vi "Test NI-Scope Performance.vi"() -> ()   [LabVIEW 2016]
uses:
  NI-Scope Lock-in Driver/NI-Scope Lock-in Configuration.ctl
  Instruments/Temperature Controller Driver/T controller configuration.ctl
  NI-Scope Lock-in Driver/NI-Scope Lock-in Driver.lvclass
  C:/github/NHMFL_Core/Libraries/Instruments/Pulse Driver/Pulse Driver.lvclass
  C:/github/NHMFL_Core/Libraries/NI-DAQ/NI-Scope Digitizer/Ni-Scope Digitizer.lvclass
  Instruments/Cryo-con/Cryo-Con Driver/Cryo-Con Driver.lvclass
  C:/github/NHMFL_Core/Libraries/Instruments/VISA Instrument/VISA Instrument.lvclass
  C:/github/NHMFL_Core/Libraries/Instruments/Temperature Controller Driver/Temperature Controller Driver.lvclass
  C:/github/NHMFL_Core/Libraries/Instruments/Instrument Driver/Instrument Driver.lvclass
  Instruments/Pulse Driver/Pulse Driver.lvclass/Pulse Driver.ctl
  Ni-Scope Digitizer.lvclass/Ni-Scope Digitizer.ctl
  Instruments/VISA Instrument/VISA Instrument.lvclass/VISA Instrument.ctl
  Instruments/Instrument Driver/Instrument Driver.lvclass/Instrument Driver.ctl
  Instruments/VISA Instrument/Write VISA resource.vi
  Instruments/Instrument Driver/Write Recorder name.vi
  Instruments/Pulse Driver/Write tdms file.vi
  Write Device name.vi
  Write Fetch Relative To.vi
  Instruments/Pulse Driver/Write Samples per read.vi
  Instruments/Temperature Controller Driver/Write T controller configuration.vi
  Instruments/Results/Acquired Result/Acquired Result.lvclass
panel:
  in  "T controller configuration":T1={"Record Channels"=["A"], "Add raw signal"=FALSE, "New set point"=0.0}
  in  "Cryocon VISA resource":refnum<visa-resource-name>="COM4"
  out "File Path Control":path
  out "Waveform Chart":dynamicdata(graph)
  in  "milliseconds to wait":u32=1000
  in  "Configuration":T2={"Points per sine wave"=64, "Rate"=4096012.1154785156, "Re-name channels"=["I", "Va", "Vc1", "Vc2"], "Active channels"="2", "Ranges"=[10.0], "Sync on trigger"=TRUE, "R-Q"=FALSE} {"Ranges" format="%#_6pV"; "Rate" format="%#_8pHz"}
  in  "Device name":refnum<k15>="5105-PCI"
  in  "Stop Button":bool
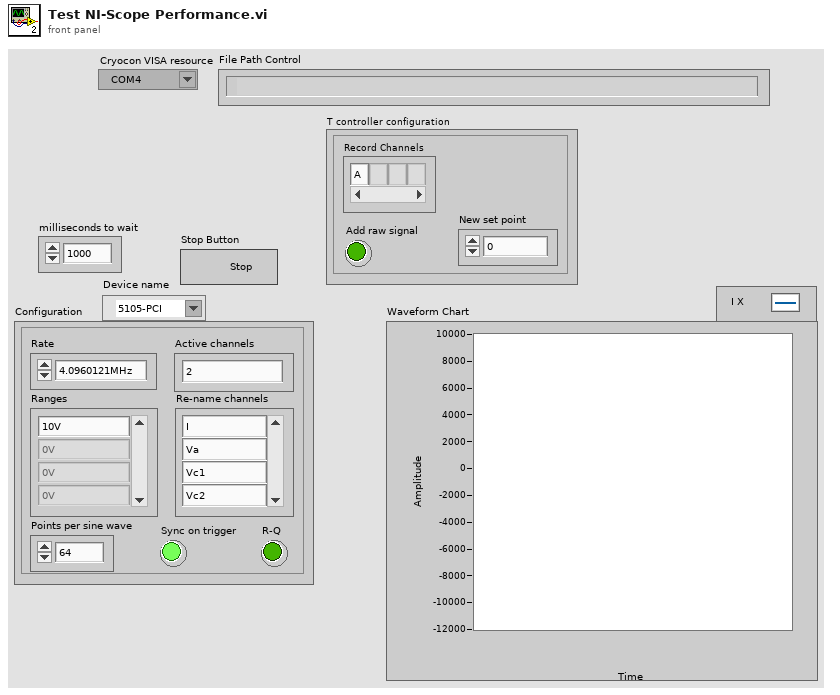
[diagram p1: front panel]
types:
  T1 = typedef "T controller configuration.ctl" = cluster{"Record Channels":string[], "Add raw signal":bool, "New set point":dbl}
  T2 = typedef "NI-Scope Lock-in Configuration.ctl" = cluster{"Points per sine wave":i32, "Rate":dbl, "Re-name channels":string[], "Active channels":string, "Ranges":dbl[], "Sync on trigger":bool, "R-Q":bool}
  T3 = enum16{"open", "open or create", "create or replace", "create", "open (read-only)"}
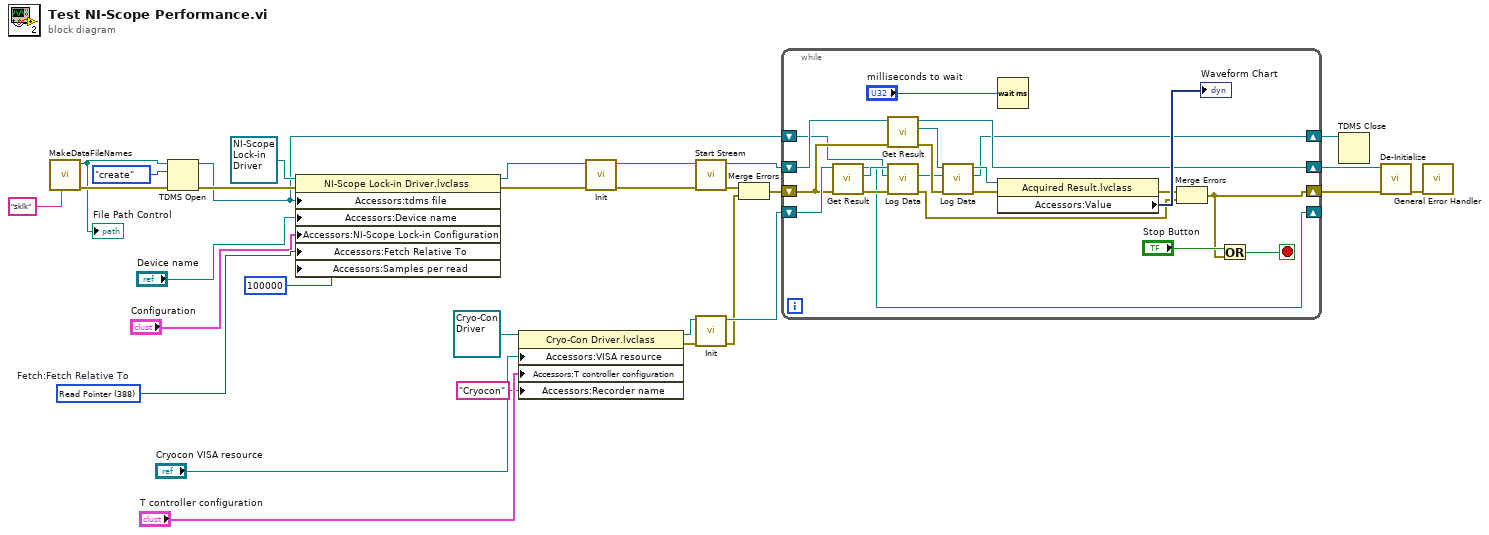
[diagram p0: block diagram]
diagram:
  w28 = 388 items=["Start"=482, "Trigger"=483, "Pretrigger"=477, "Now"=481, "Read Pointer"=388]  # Fetch:Fetch Relative To
  n1 = call "MakeDataFileNames.vi"("File Prefix"="sklk") -> ("Error Out"=w22:errorcluster, "Data File  Path"=w18:path)  [unwired: 7 in, 2 out]
  "File Path Control" <- w18
  n2 = TDMS Open(8:w22, 10:T3."create" ("operation (0:open)"), 11:w18) -> (0:w21:errorcluster, 3:w13:refnum<k34>)  [unwired: 4 in]
  n3 = property class="NI-Scope Lock-in Driver.lvclass"(reference=refnum<class "NI-Scope Lock-in Driver.lvclass"> refnum ("NI-Scope Lock-in Driver.lvclass"), error in=w21, "Accessors:tdms file"=w13, "Accessors:Device name"="Device name", "Accessors:NI-Scope Lock-in Configuration"="Configuration", "Accessors:Fetch Relative To"=w28, "Accessors:Samples per read"=100000 ("Samples per read")) -> (reference out=w29:refnum<class "NI-Scope Lock-in Driver.lvclass">, error out=w10:errorcluster)
  n4 = property class="Cryo-Con Driver.lvclass"(reference=refnum<class "Cryo-Con Driver.lvclass"> refnum ("Cryo-Con Driver.lvclass"), "Accessors:VISA resource"="Cryocon VISA resource", "Accessors:T controller configuration"="T controller configuration", "Accessors:Recorder name"="Cryocon" ("Recorder name")) -> (reference out=w6:refnum<class "Cryo-Con Driver.lvclass">, error out=w4:errorcluster)  [unwired: 1 in]
  n5 = call-dynamic "Init.vi"("error in (no error)"=w10, "Instrument Driver in"=w29) -> ("error out"=w15:errorcluster, "Instrument Driver out"=w17:refnum<class "NI-Scope Lock-in Driver.lvclass">)  [unwired: 7 in, 1 out]
  n6 = call-dynamic "Start Stream.vi"("error in (no error)"=w15, "Ni-Scope Digitizer in"=w17) -> ("error out"=w14:errorcluster, "Ni-Scope Digitizer out"=w16:refnum<class "NI-Scope Lock-in Driver.lvclass">)  [unwired: 8 in]
  n7 = call-dynamic "Init.vi"("error in (no error)"=w4, "Instrument Driver in"=w6) -> ("error out"=w3:errorcluster, "Instrument Driver out"=w5:refnum<class "Cryo-Con Driver.lvclass">)  [unwired: 7 in, 1 out]
  n8 = Merge Errors(w14, w3) -> (w9:errorcluster)
  n9 = while {
    shift-right: [w45] -> w26
    shift-left: w16 -> [w48]
    shift-right: [w31] -> w27
    shift-left: w9 -> [w39]
    shift-right: [w36] -> w8
    shift-left: w13 -> [w35]
    shift-right: [w32] -> _
    shift-left: w5 -> [w40]
    stop <- w49 stop-if-true
    n10 = call-dynamic "Get Result.vi"("error in (no error)"=w39, "Simple VISA Reader Driver in"=w40) -> ("error out"=w37:errorcluster, "Result"=w38:refnum<class "Acquired Result.lvclass">, "Simple VISA Reader Driver out"=w32:refnum<class "Cryo-Con Driver.lvclass">)  [unwired: 7 in]
    n11 = call-dynamic "Get Result.vi"("error in (no error)"=w39, "NI-Scope Lock-in Driver in"=w48) -> ("error out"=w43:errorcluster, "Result"=w44:refnum<class "Acquired Result.lvclass">, "NI-Scope Lock-in Driver out"=w45:refnum<class "NI-Scope Lock-in Driver.lvclass">)  [unwired: 7 in]
    n12 = call-dynamic "Log Data.vi"("error in (no error)"=w37, "tdms file"=w35, "Acquired Result in"=w38) -> ("error out"=w33:errorcluster, "tdms file out"=w34:refnum<k34>)  [unwired: 6 in, 1 out]
    n13 = call-dynamic "Log Data.vi"("error in (no error)"=w43, "tdms file"=w34, "Acquired Result in"=w44) -> ("error out"=w42:errorcluster, "tdms file out"=w36:refnum<k34>, "Acquired Result out"=w41:refnum<class "Acquired Result.lvclass">)  [unwired: 6 in]
    n14 = Wait (ms)(milliseconds to wait="milliseconds to wait") -> ()  [unwired: 1 out]
    n15 = property class="Acquired Result.lvclass"(reference=w41, error in=w42) -> (error out=w46:errorcluster, "Accessors:Value"=→"Waveform Chart":dynamicdata)  [unwired: 1 out]
    n16 = Merge Errors(w46, w33) -> (w31:errorcluster)
    n17 = Or(x="Stop Button", y=w31) -> (x .or. y?=w49:bool)
  }
  n18 = TDMS Close(11:w8) -> ()  [unwired: 1 in, 2 out]
  n19 = call-dynamic "De-Initialize.vi"("error in (no error)"=w27, "Ni-Scope Digitizer in"=w26) -> ("error out"=w25:errorcluster)  [unwired: 8 in, 1 out]
  n20 = call <vilib>:"General Error Handler.vi"("error in (no error)"=w25) -> ()  [unwired: 10 in, 5 out]
